vi "test17-RegisterStatesFromNonCSM_State.vi"(8 "error in (no error)":errorcluster, 11 "TestCase in":refnum<class "testcase-CSMStatusStateRegisterUnregister.lvclass">) -> (0 "error out":errorcluster, 3 "TestCase out":refnum<class "testcase-CSMStatusStateRegisterUnregister.lvclass">)   [LabVIEW 2017, in "testcase-CSMStatusStateRegisterUnregister.lvclass"]
uses:
  testcase-CSMStatusStateRegisterUnregister.lvclass
  <vilib>/addons/_JKI Toolkits/VI Tester/TestCase.llb/TestCase.lvclass
  src/user.lib/_NEVSTOP/Communicable State Machine(CSM)/Communicable State Machine.lvlib
  C:/Program Files (x86)/National Instruments/LabVIEW 2017/vi.lib/addons/_JKI Toolkits/VI Tester/TestCase.llb/TestCase.lvclass
panel:
  out "error out 3":errorcluster
  out "error out 2":errorcluster
  out "LoopCount":i32
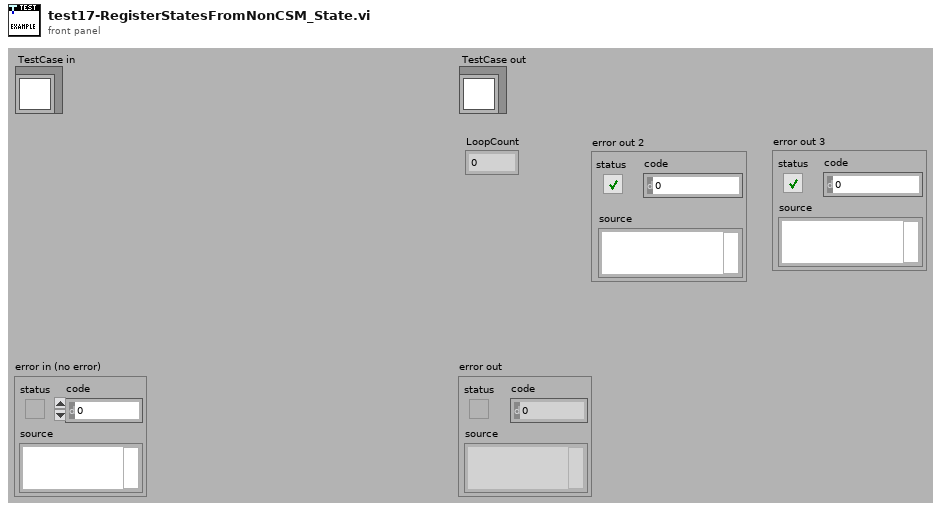
[diagram p1: front panel]
types:
  T1 = cluster{"ModuleName":string, "Status":string, "Arguments":string}
  T2 = cluster{"cluster":cluster{"ModuleName":string, "Status":string, "Arguments":string}}
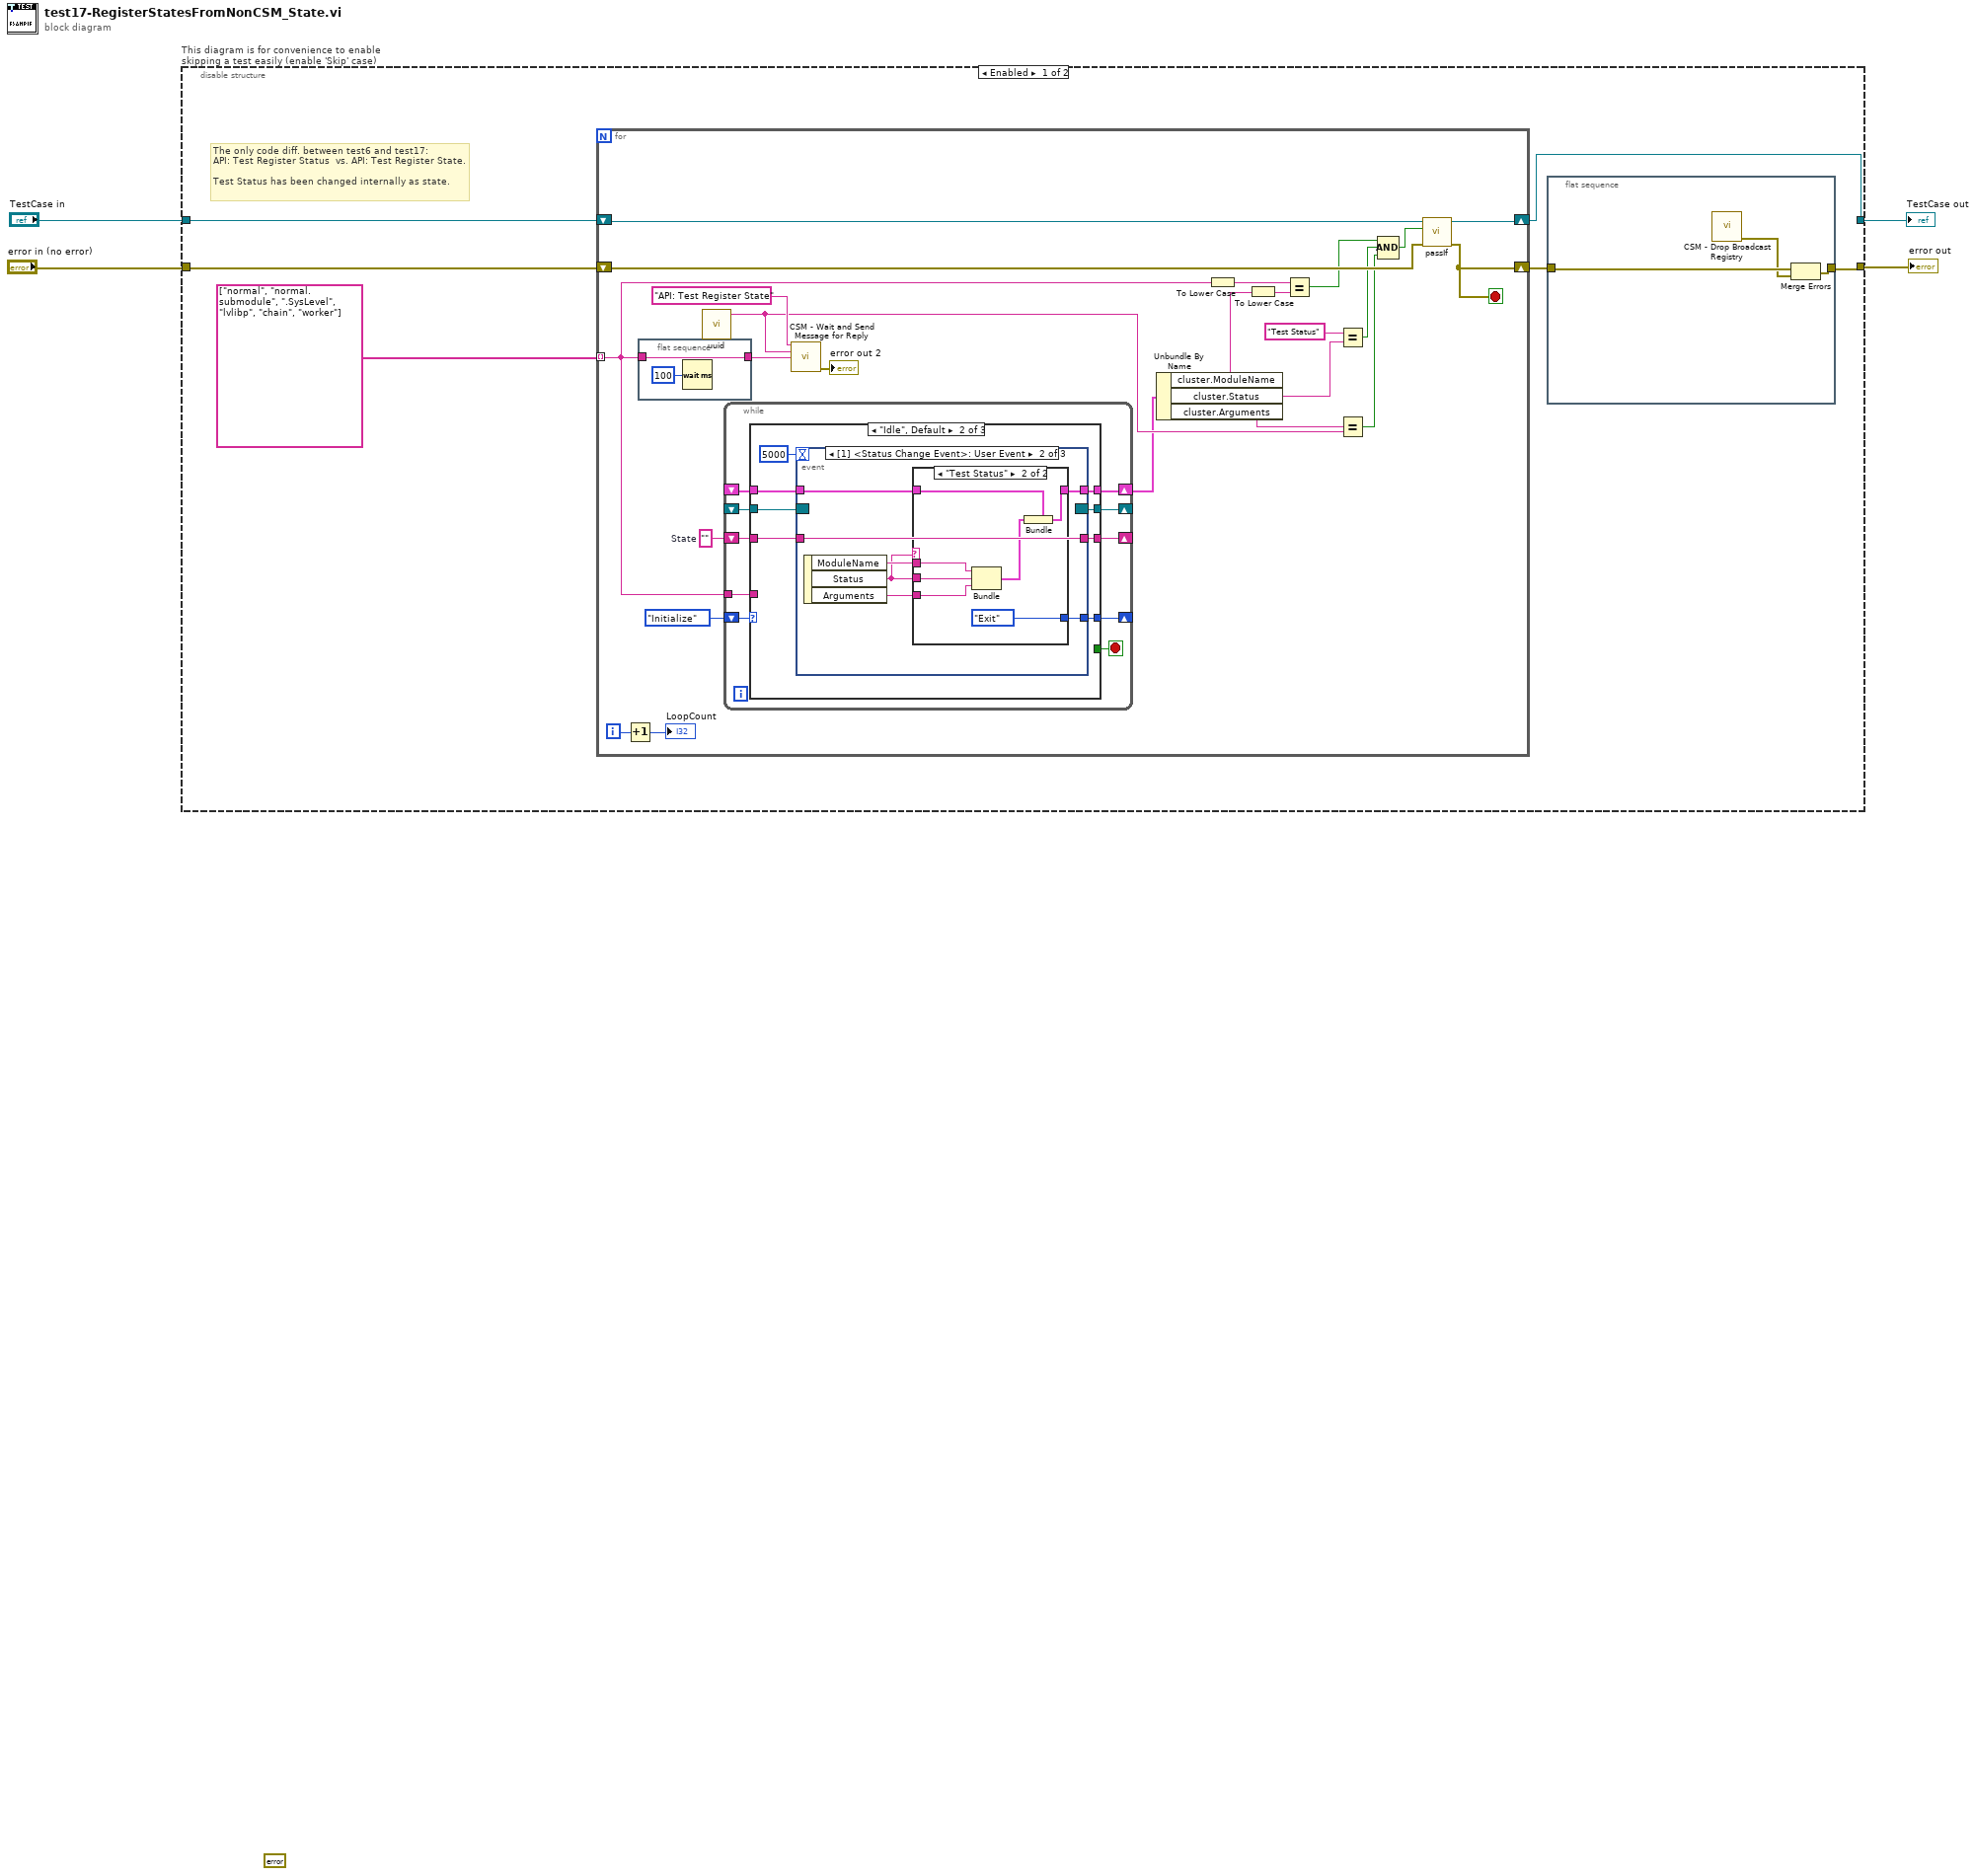
[diagram p0: block diagram]
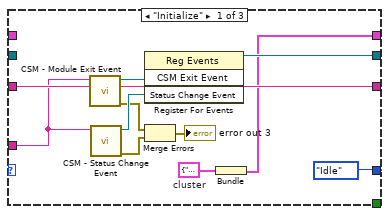
[diagram p2: hidden frame]
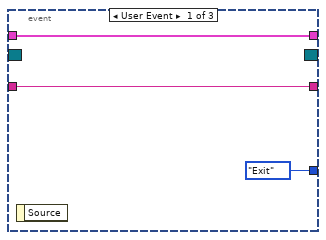
[diagram p3: hidden frame]
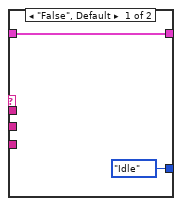
[diagram p4: hidden frame]
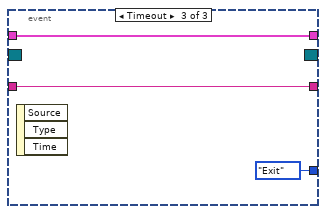
[diagram p5: hidden frame]
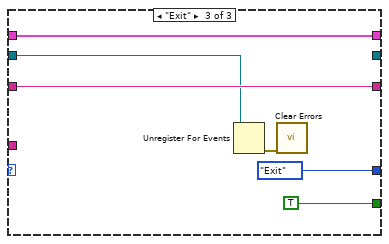
[diagram p6: hidden frame]
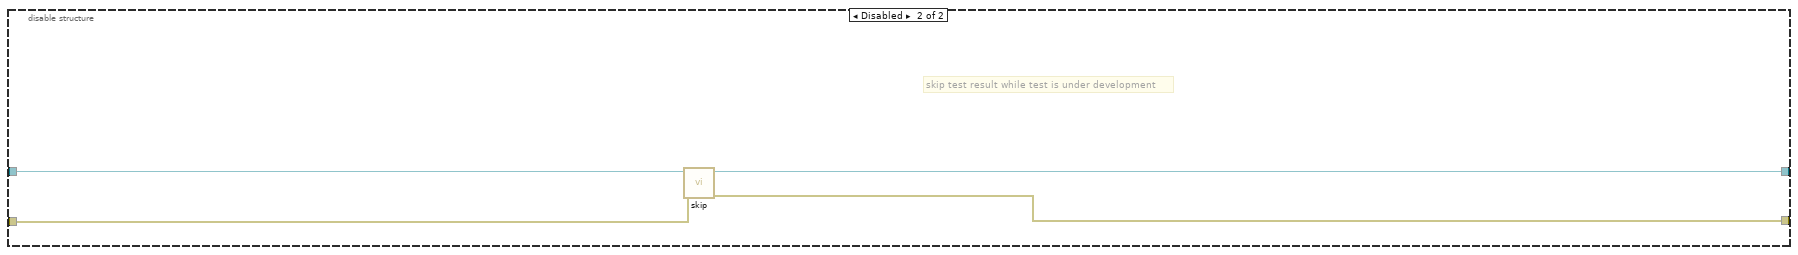
[diagram p7: hidden frame]
diagram:
  (unwired) errorcluster {"status"=FALSE, "code"=0, "source"=""} ("error out")
  n1 = disable-structure "This diagram is for convenience to enable skipping a test easily (enable 'Skip' case)" shown="Enabled" {
    disable-tunnel: "TestCase in" -> [w10 w100]
    disable-tunnel: [w6 w98] -> w2
    disable-tunnel: [w5 w99] -> w1
    disable-tunnel: "error in (no error)" -> [w9 w97]
    frame Enabled {
      # "The only code diff. between test6 and test17:\nAPI: Test Register Status  vs. API: Test Register State.\n\nTest Status has been changed internally as state."
      n2 = for {
        shift-right: [w28] -> w6
        shift-left: w10 -> [w29]
        shift-right: [w19] -> w7
        shift-left: w9 -> [w27]
        tunnel: string[] ["normal", "normal.submodule", ".SysLevel", "lvlibp", "chain", "worker"] -> [w17] mode=indexing
        i -> [w22]
        stop <- w19 stop-if-true
        w36 = ""  # State
        n3 = Increment(x=w22) -> (x+1=→"LoopCount":i32)
        n4 = flat-sequence {
          tunnel: w17 -> [w39]
          tunnel: [w39] -> w34
          frame #0 {
            n5 = Wait (ms)(milliseconds to wait=u32 100) -> ()  [unwired: 1 out]
          }
        }
        n6 = call "uuid.vi"() -> ("UUID"=w31:string)  [unwired: 11 in]
        n7 = while {
          shift-right: [w48] -> _
          shift-left: enum16{"Idle", "Initialize", "Exit"}."Initialize" -> [w49]
          shift-right: [w45] -> _
          shift-left: w36 -> [w46]
          shift-right: [w44] -> _
          shift-left: _ -> [w43]
          shift-right: [w42] -> w18
          shift-left: _ -> [w41]
          tunnel: w17 -> [w40]
          stop <- w47 stop-if-true
          n8 = case shown="\"Idle\", Default" w49 {
            tunnel: [enum16{"Idle", "Initialize", "Exit"}."Idle" w68 enum16{"Idle", "Initialize", "Exit"}."Exit"] -> w48
            tunnel: [_ _ TRUE] -> w47
            tunnel: w46 -> [w59 w66 w94]
            tunnel: [w59 w67 w94] -> w45
            tunnel: [w57 w64 _] -> w44
            tunnel: w43 -> [_ w65 w93]
            tunnel: [w56 w62 w91] -> w42
            tunnel: w41 -> [_ w63 w91]
            tunnel: w40 -> [w54 _ _]
            frame "Initialize" {
              w53 = T1 {"ModuleName"="", "Status"="", "Arguments"=""}  # cluster
              n9 = call "CSM - Module Exit Event.vi"("Name (\"\" to Use UUID) In"=w54) -> ("error out"=w52:errorcluster, "CSM Exit Event"=w58:refnum<user-event>)  [unwired: 8 in, 1 out]
              n10 = call "CSM - Status Change Event.vi"("CSM Module"=w54) -> ("error out"=w51:errorcluster, "Status Change Event"=w55:refnum<user-event>)  [unwired: 8 in, 1 out]
              n11 = register-events(w58, w55) -> (reference out=w57:refnum<event-registration>)  [unwired: 2 in, 1 out]
              n12 = Merge Errors(w52, w51) -> (→"error out 3":errorcluster)
              n13 = Bundle("cluster"=w53) -> (w56:T2)  [unwired: 1 in]
            }
            frame "Idle", Default {
              n14 = event shown="[1] <Status Change Event>: User Event" {
                selector: w65 -> [_ _ _]
                dyn-events: [_ _ _] -> w64
                timeout: 5000 -> [_ _ _]
                tunnel: [enum16{"Idle", "Initialize", "Exit"}."Exit" w77 enum16{"Idle", "Initialize", "Exit"}."Exit"] -> w68
                tunnel: w66 -> [w71 w78 w90]
                tunnel: [w71 w78 w90] -> w67
                tunnel: w63 -> [w69 w74 w89]
                tunnel: [w69 w73 w89] -> w62
                event User Event {
                  n15 = event-data() -> ()  [unwired: 1 in, 1 out]
                }
                event User Event {
                  n16 = event-data() -> ("ModuleName"=w76:string, "Status"=w72:string, "Arguments"=w75:string)  [unwired: 1 in]
                  n17 = case shown="\"Test Status\"" w72 {
                    tunnel: [enum16{"Idle", "Initialize", "Exit"}."Idle" enum16{"Idle", "Initialize", "Exit"}."Exit"] -> w77
                    tunnel: w76 -> [_ w86]
                    tunnel: w72 -> [_ w85]
                    tunnel: w75 -> [_ w84]
                    tunnel: w74 -> [w80 w83]
                    tunnel: [w80 w81] -> w73
                    frame "False", Default {
                    }
                    frame "Test Status" {
                      n18 = Bundle("ModuleName"=w86, "Status"=w85, "Arguments"=w84) -> (w82:T1)  [unwired: 1 in]
                      n19 = Bundle(cluster=w83, "cluster"=w82) -> (w81:T2)
                    }
                  }
                }
                event Timeout {
                  n20 = event-data() -> ()  [unwired: 1 in, 3 out]
                }
              }
            }
            frame "Exit" {
              n21 = Unregister For Events(event registration refnum=w93) -> (error out=w92:errorcluster)  [unwired: 1 in]
              n22 = call <vilib>:"Clear Errors.vi"("error in (no error)"=w92) -> ()  [unwired: 5 in, 2 out]
            }
          }
        }
        n23 = call "CSM - Wait and Send Message for Reply.vi"("State"="API: Test Register State", "Arguments (\"\")"=w31, "Target Module"=w34) -> ("error out"=→"error out 2":errorcluster)  [unwired: 10 in, 2 out]
        n24 = Unbundle By Name(w18) -> ("cluster.ModuleName"=w15:string, "cluster.Status"=w32:string, "cluster.Arguments"=w30:string)
        n25 = To Lower Case(string=w17) -> (all lower case string=w16:string)
        n26 = To Lower Case(string=w15) -> (all lower case string=w14:string)
        n27 = Equal?(x=w16, y=w14) -> (x = y?=w26:bool)
        n28 = Equal?(x="Test Status" ("State"), y=w32) -> (x = y?=w25:bool)
        n29 = Equal?(x=w30, y=w31) -> (x = y?=w24:bool)
        n30 = Compound Arithmetic op=AND(w26, w25, w24) -> (w23:bool)
        n31 = call-dynamic "passIf.vi"("error in (no error)"=w27, "pass"=w23, "TestCase in"=w29) -> ("error out"=w19:errorcluster, "TestCase out"=w28:refnum<class "testcase-CSMStatusStateRegisterUnregister.lvclass">)  [unwired: 7 in]
      }
      n32 = flat-sequence {
        tunnel: w7 -> [w13]
        tunnel: [w12] -> w5
        frame #0 {
          n33 = call "CSM - Drop Broadcast Registry.vi"() -> ("error out"=w11:errorcluster)  [unwired: 15 in]
          n34 = Merge Errors(w13, w11) -> (w12:errorcluster)
        }
      }
    }
    frame Disabled {
      # "skip test result while test is under development"
      n35 = call <vilib>:"skip.vi"("error in (no error)"=w97, "TestCase in"=w100) -> ("error out"=w99:errorcluster, "TestCase out"=w98:refnum<class "testcase-CSMStatusStateRegisterUnregister.lvclass">)  [unwired: 8 in]
    }
  }
  "error out" <- w1
  "TestCase out" <- w2
